vi "Hvtronc(asp).vi"(8 "Q":dbl, 9 "d1":dbl, 10 "rug(1)":dbl, 11 "lungh(1)":dbl) -> (2 "Hvtronch(1)":dbl, 3 "lambda(1)":dbl)   [LabVIEW 2016]
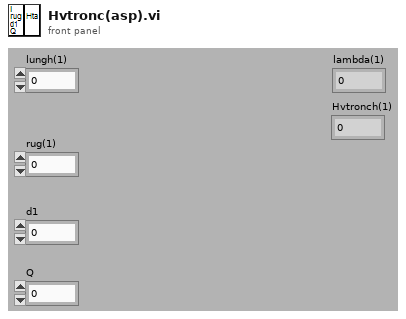
[diagram p1: front panel]
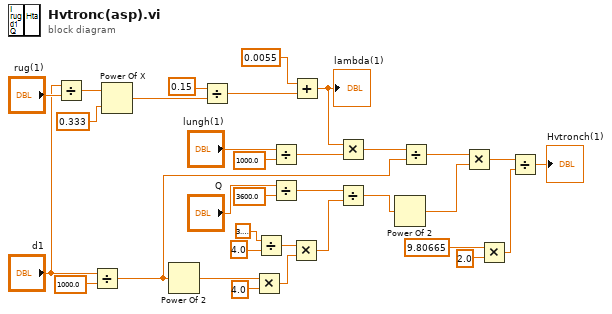
[diagram p0: block diagram]
diagram:
  n1 = Divide(x="d1", y="rug(1)") -> (x/y=w32:dbl)
  n2 = Divide(x="d1", y=1000.0) -> (x/y=w19:dbl)
  n3 = Power Of X(1:0.333 ("x"), 2:w32) -> (0:w28:dbl)
  n4 = Power Of 2(x=w19) -> (2^x=w18:dbl)
  n5 = Divide(x=0.15, y=w28) -> (x/y=w27:dbl)
  n6 = Multiply(x=w18, y=4.0) -> (x*y=w13:dbl)
  n7 = Divide(x=3.141592653589793, y=4.0) -> (x/y=w14:dbl)
  n8 = Divide(x="lungh(1)", y=1000.0) -> (x/y=w9:dbl)
  n9 = Divide(x="Q", y=3600.0) -> (x/y=w7:dbl)
  n10 = Multiply(x=w14, y=w13) -> (x*y=w12:dbl)
  n11 = Add(x=0.0055, y=w27) -> (x+y=w10:dbl)
  "lambda(1)" <- w10
  n12 = Multiply(x=w10, y=w9) -> (x*y=w22:dbl)
  n13 = Divide(x=w7, y=w12) -> (x/y=w11:dbl)
  n14 = Power Of 2(x=w11) -> (2^x=w6:dbl)
  n15 = Divide(x=w22, y=w19) -> (x/y=w8:dbl)
  n16 = Multiply(x=w8, y=w6) -> (x*y=w3:dbl)
  n17 = Multiply(x=9.80665, y=2.0) -> (x*y=w2:dbl)
  n18 = Divide(x=w3, y=w2) -> (x/y=→"Hvtronch(1)":dbl)
